vi "Display Data.vi"(8 "Error In":errorcluster, 11 "String in":refnum<class "String.lvclass">) -> (0 "Error Out":errorcluster, 3 "String out":refnum<class "String.lvclass">)   [LabVIEW 2020, in "String.lvclass"]
doc: "The method displays the received data of string data type."
uses:
  String.lvclass
panel:
  out "String Data":string
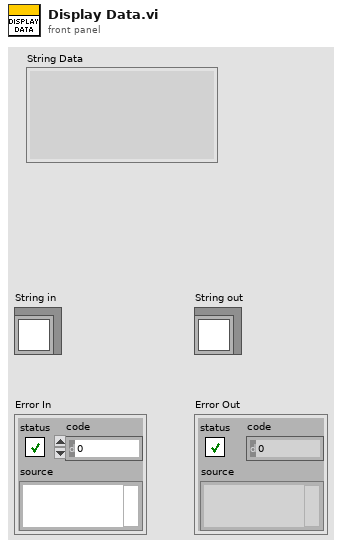
[diagram p1: front panel]
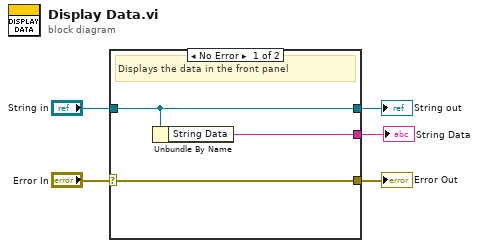
[diagram p0: block diagram]
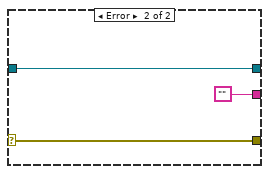
[diagram p2: hidden frame]
diagram:
  n1 = case shown="No Error" "Error In" {
    selector: "Error In" -> [w8 w11]
    tunnel: [w8 w11] -> w4
    tunnel: [w7 w10] -> w2
    tunnel: "String in" -> [w7 w10]
    tunnel: [w6 "" ("String Data")] -> w1
    frame No Error {
      # "Displays the data in the front panel"
      n2 = Unbundle By Name(w7) -> ("String Data"=w6:string)
    }
    frame Error {
    }
  }
  "Error Out" <- w4
  "String out" <- w2
  "String Data" <- w1
